vi "Logistic Moments.vi"(9 "b":dbl=1.0, 10 "a":dbl=1.0) -> (0 "error":i32, 2 "variance":dbl=3.289868133696453, 3 "mean":dbl=1.0)   [LabVIEW 2020, in "NI_Gmath.lvlib"]
doc: "Returns the expected mean and variance of the random variate X, where X describes the selected distribution type. You must manually select the polymorphic instance to use."
uses:
  <vilib>/gmath/NI_Gmath.lvlib
  <vilib>/gmath/statdist.llb/st_error_code.ctl
panel:
  # "Logistic Moments"
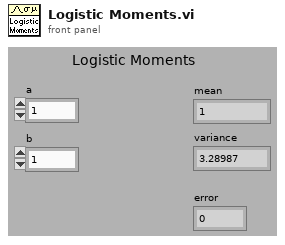
[diagram p1: front panel]
types:
  T1 = typedef "NI_Gmath.lvlib/st_error_code.ctl" = i32
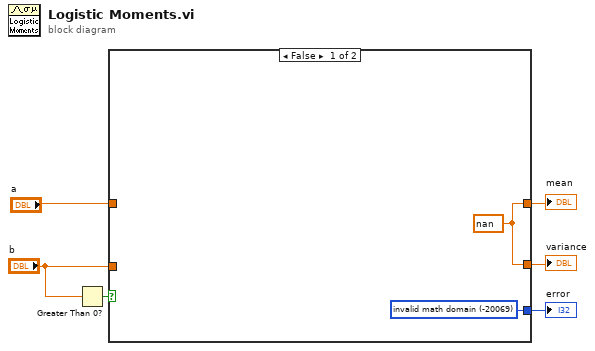
[diagram p0: block diagram]
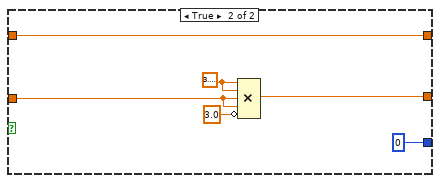
[diagram p2: hidden frame]
diagram:
  n1 = Greater Than 0?(x="b") -> (x > 0?=w3:bool)
  n2 = case shown="False" w3 {
    tunnel: [w8 0 ("invalid math domain")] -> w4
    tunnel: [w7 w13] -> w5
    tunnel: [w7 w9] -> w6
    tunnel: "a" -> [_ w13]
    tunnel: "b" -> [_ w11]
    frame False {
      w8 = T1 -20069 items=["invalid math domain"=-20069, "Fourier interpolation size m >= n"=-20070, "empty array"=-20003] ("stat interp error code")
      w7 = nan
    }
    frame True {
      w12 = 3.141592653589793
      n3 = Compound Arithmetic op=MULTIPLY(w12, w12, w11, w11, invert 3.0 ("value")) -> (w9:dbl)
    }
  }
  "mean" <- w5
  "error" <- w4
  "variance" <- w6
